vi "StateDrivebase.vi"(1 "Master State":string) -> ()   [LabVIEW 2019]
doc: "This VI performs all of the calculations and decisions related to the swerve drive. Driver profiles are tuned from this front panel."
uses:
  <vilib>/Rock Robotics/WPI/DriverStation/WPI_DriverStationRobotMode2.ctl
  dsinstructions.vi
  constants.vi
  dsdata.vi
  sensors.vi
  outputs.vi
panel:
  in  "PID Tuning Heading Lock":T1={"Kp"=0.00045, "Ki"=0.0, "Kd"=0.0, "N-Diff"=3, "N-Int"=10, "Int Error Window"=90.0, "Max Ouput"=1.0, "Min Output"=-1.0, "Square Derivative"=FALSE, "N-Prop"=5} {"N-Prop" min=1; "Int Error Window" min=0.0; "N-Int" min=2; "N-Diff" min=2; "Kd" min=0.0; "Ki" min=0.0; "Kp" min=0.0}
  in  "Driver Profiles":T2(array[cluster])=[{"Strafe Deadband"=0.08, "Strafe Scaling"=2.0, "Strafe Maximum"=1.0, "Rotation Deadband"=0.15, "Rotation Scaling"=2.5, "Rotation Maximum"=1.0}, {"Strafe Deadband"=0.08, "Strafe Scaling"=2.0, "Strafe Maximum"=1.0, "Rotation Deadband"=0.15, "Rotation Scaling"=2.5, "Rotation Maximum"=1.0}, {"Strafe Deadband"=0.08, "Strafe Scaling"=2.0, "Strafe Maximum"=1.0, "Rotation Deadband"=0.15, "Rotation Scaling"=2.5, "Rotation Maximum"=1.0}, {"Strafe Deadband"=0.08, "Strafe Scaling"=2.0, "Strafe Maximum"=1.0, "Rotation Deadband"=0.03, "Rotation Scaling"=2.5, "Rotation Maximum"=1.0}, {"Strafe Deadband"=0.08, "Strafe Scaling"=2.0, "Strafe Maximum"=1.0, "Rotation Deadband"=0.15, "Rotation Scaling"=2.5, "Rotation Maximum"=1.0}, {"Strafe Deadband"=0.08, "Strafe Scaling"=2.0, "Strafe Maximum"=1.0, "Rotation Deadband"=0.15, "Rotation Scaling"=2.5, "Rotation Maximum"=1.0}, {"Strafe Deadband"=0.08, "Strafe Scaling"=2.0, "Strafe Maximum"=0.5, "Rotation Deadband"=0.15, "Rotation Scaling"=2.5, "Rotation Maximum"=0.3}] {"Rotation Maximum" min=0.3 max=1.0 scale=0.3..1.0; "Rotation Scaling" min=1.0 max=4.0 scale=1.0..4.0; "Rotation Deadband" min=0.0 max=0.25 scale=0.0..0.25; "Strafe Maximum" min=0.3 max=1.0 scale=0.3..1.0; "Strafe Scaling" min=1.0 max=4.0 scale=1.0..4.0; "Strafe Deadband" min=0.0 max=0.25 scale=0.0..0.25}
  in  "Deceleration Hysteresis (ms)":u32=1
  out "Heading Control":bool
  in  "Heading Lock Strafe Deadband (ft/s)":dbl=3.0
  in  "Manually Disable Heading Lock":bool
  in  "PID Tuning Feeder Station":T3={"Kp"=0.0045, "Ki"=0.01, "Kd"=0.0002, "N-Diff"=10, "N-Int"=10, "Int Error Window"=30.0, "Max Ouput"=1.0, "Min Output"=-1.0} {"Int Error Window" min=0.0; "N-Int" min=2; "N-Diff" min=2; "Kd" min=0.0; "Ki" min=0.0; "Kp" min=0.0}
  out "Heading Controller Summary":T4(graph)
  in  "PID Tuning Auto Targeting":T3={"Kp"=0.0045, "Ki"=0.01, "Kd"=0.0002, "N-Diff"=10, "N-Int"=10, "Int Error Window"=30.0, "Max Ouput"=1.0, "Min Output"=-1.0} {"Int Error Window" min=0.0; "N-Int" min=2; "N-Diff" min=2; "Kd" min=0.0; "Ki" min=0.0; "Kp" min=0.0}
  in  "Manual Fudge Factor (deg)":dbl=5.0
  in  "Plot Heading PID":bool
  in  "Sync Driver Profile":bool
  out "Selected Driver":string
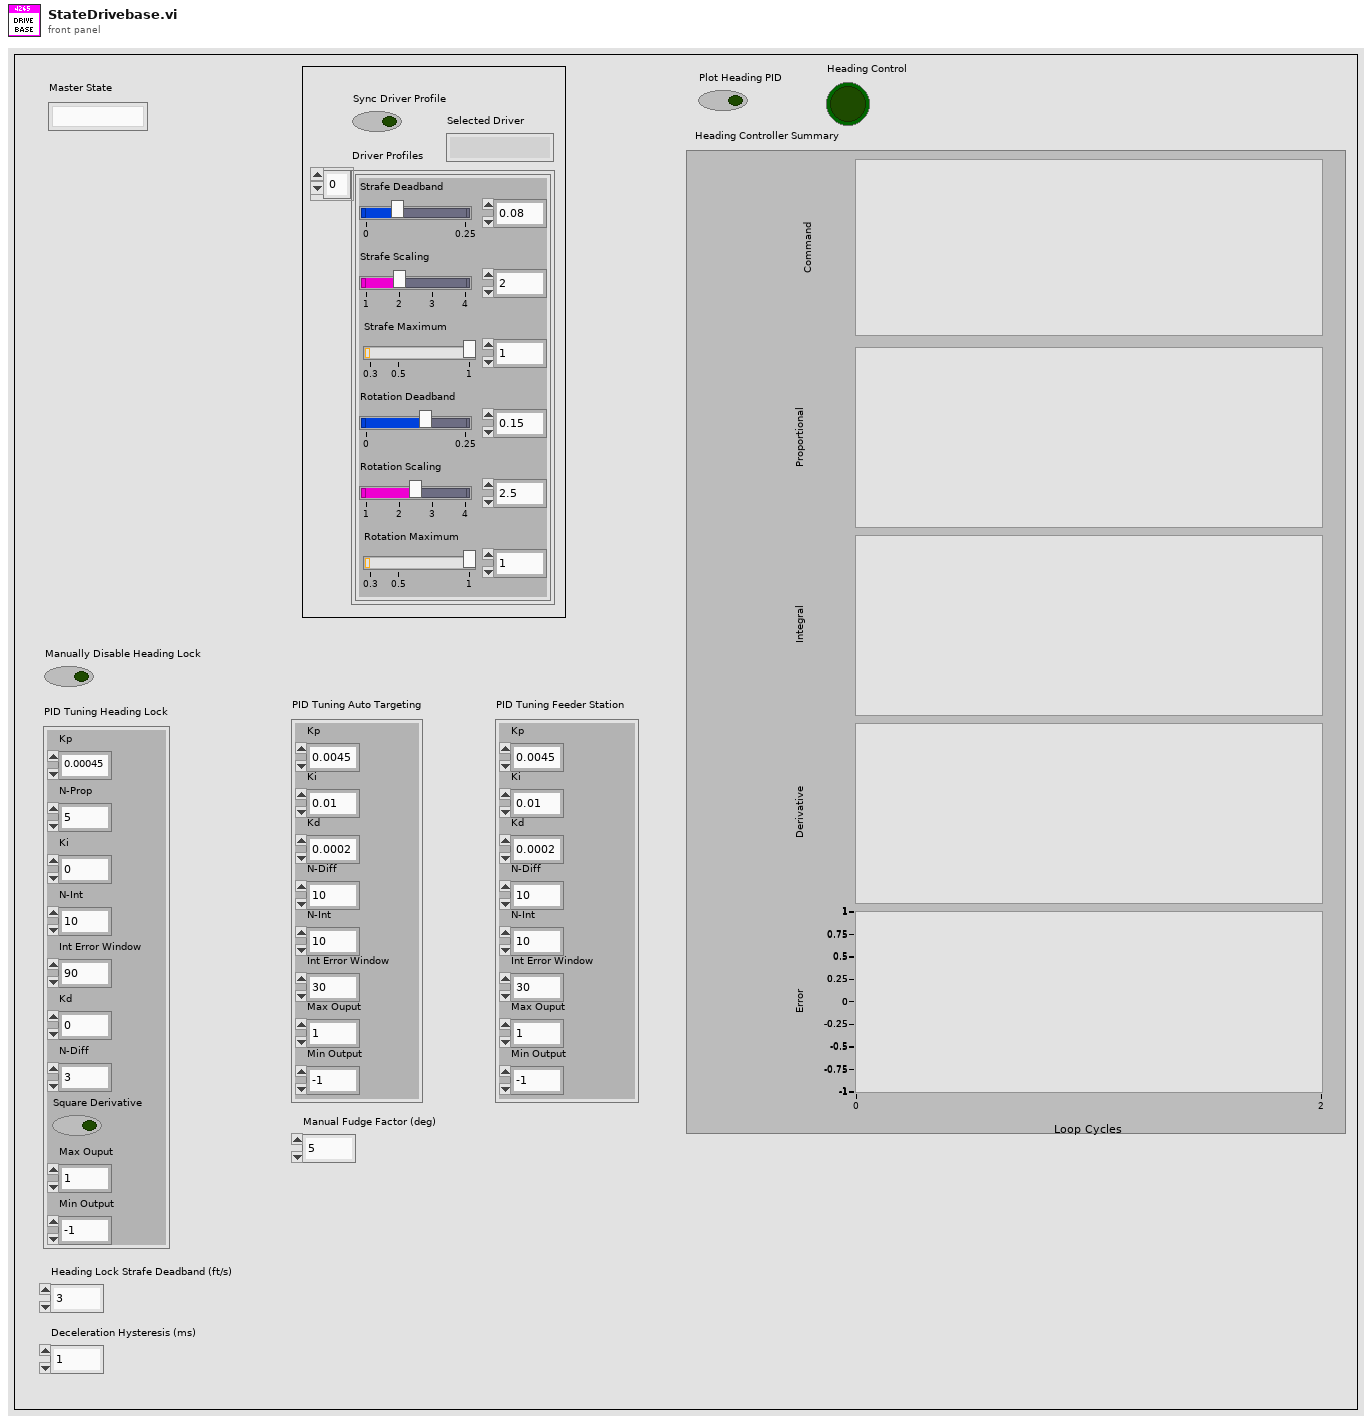
[diagram p1: front panel]
types:
  T1 = cluster{"Kp":dbl, "Ki":dbl, "Kd":dbl, "N-Diff":i32, "N-Int":i32, "Int Error Window":dbl, "Max Ouput":dbl, "Min Output":dbl, "Square Derivative":bool, "N-Prop":i32}
  T2 = cluster{"Strafe Deadband":dbl, "Strafe Scaling":dbl, "Strafe Maximum":dbl, "Rotation Deadband":dbl, "Rotation Scaling":dbl, "Rotation Maximum":dbl}[]
  T3 = cluster{"Kp":dbl, "Ki":dbl, "Kd":dbl, "N-Diff":i32, "N-Int":i32, "Int Error Window":dbl, "Max Ouput":dbl, "Min Output":dbl}
  T4 = cluster{"Command":dbl, "Proportional":dbl, "Integral":dbl, "Derivative":dbl, "Goal":dbl}
  T5 = enum16{"Driver Control", "Auto Targeting", "Feeder Station"}
  T6 = typedef "WPI_DriverStationRobotMode2.ctl" = enum16{"Autonomous Disabled", "Autonomous Enabled", "Teleop Disabled", "Teleop Enabled", "Disconnected", "Finish", "Test Disabled", "Test Enabled", "Emergency Stopped"}
  T7 = cluster{"Strafe Deadband":dbl, "Strafe Scaling":dbl, "Strafe Maximum":dbl, "Rotation Deadband":dbl, "Rotation Scaling":dbl, "Rotation Maximum":dbl}
  T8 = enum16{"Center", "Module 0", "Module 1", "Module 2", "Module 3"}
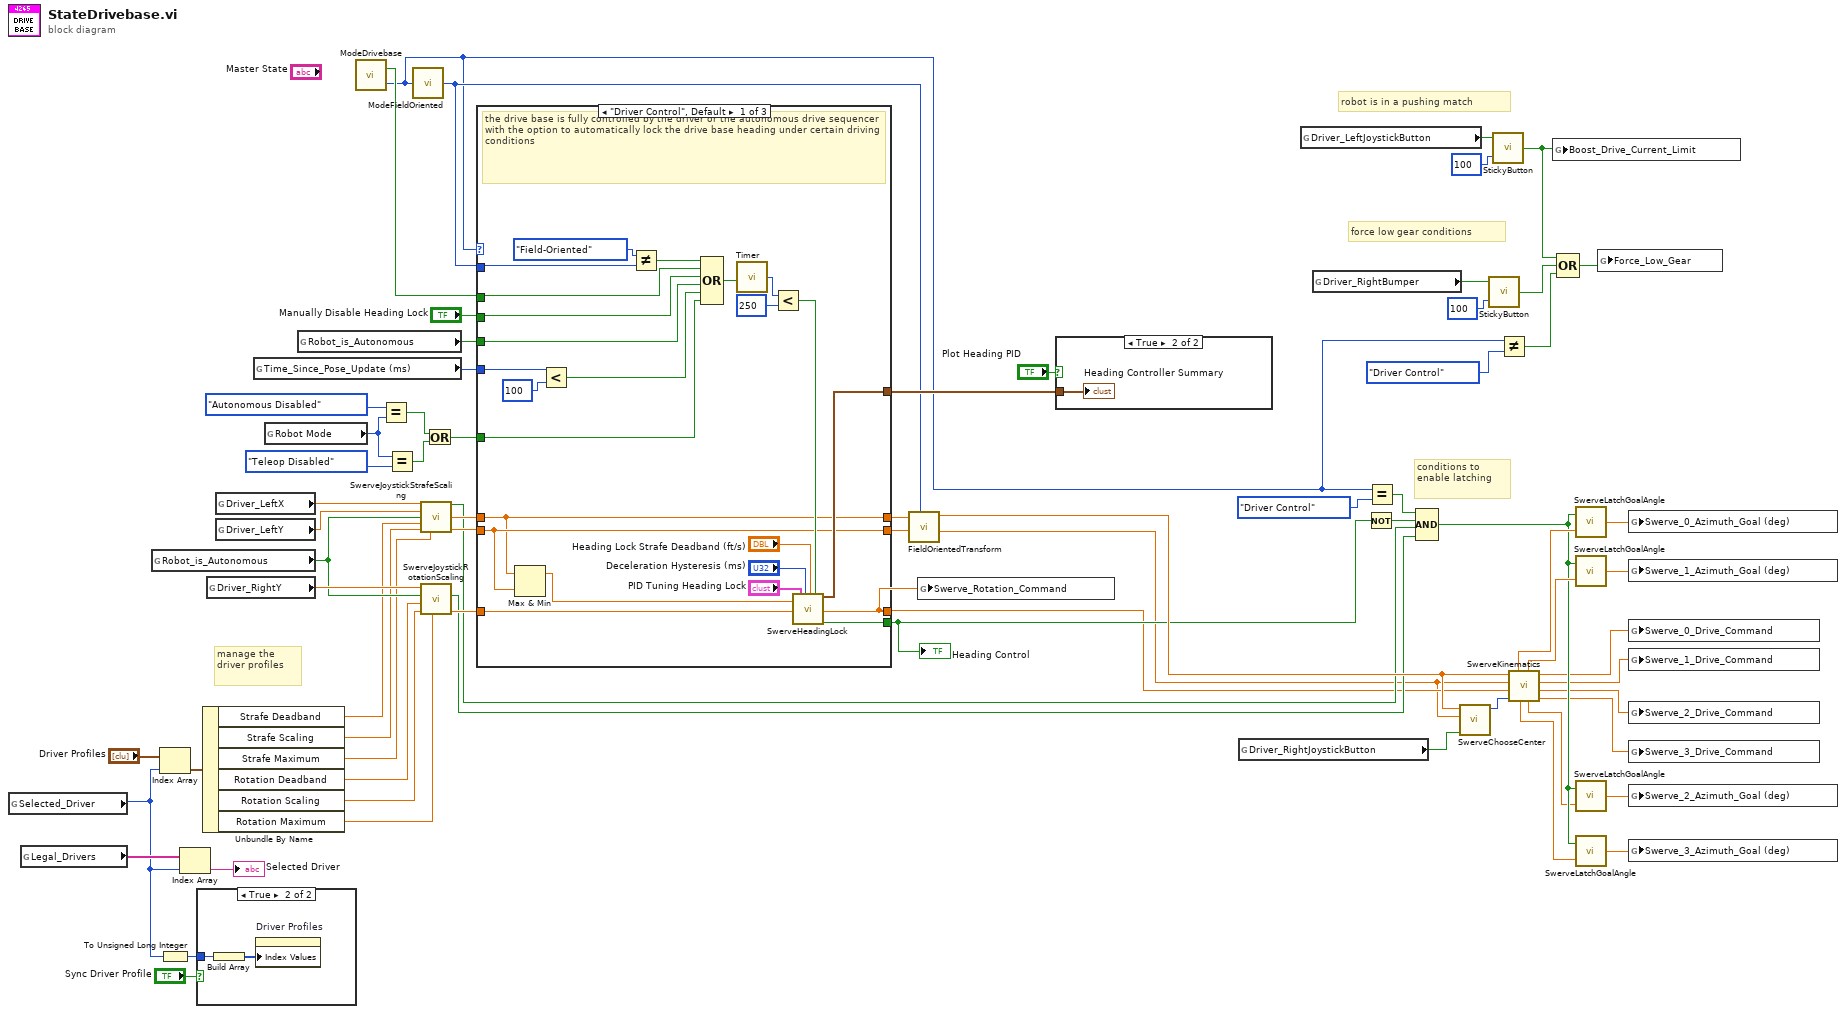
[diagram p0: block diagram]
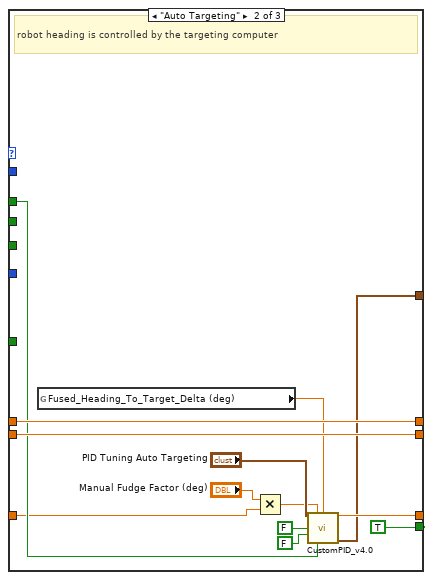
[diagram p3: hidden frame]
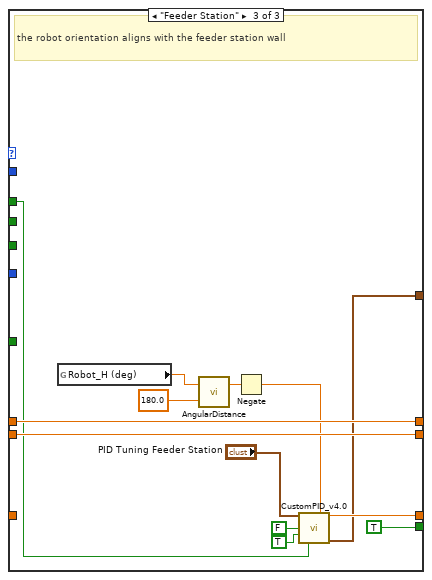
[diagram p4: hidden frame]
diagram:
  # "force low gear conditions"
  # "robot is in a pushing match"
  # "conditions to\nenable latching"
  # "manage the\ndriver profiles"
  n1 = global read "dsdata.vi" "Selected_Driver"() -> (w31:i32)
  n2 = global read "constants.vi" "Legal_Drivers"() -> (w63:string[])
  n3 = global read "dsdata.vi" "Robot_is_Autonomous"() -> (w43:bool)
  n4 = Index Array(array="Driver Profiles", index=w31) -> (element=w30:T7)
  n5 = To Unsigned Long Integer(number=w31) -> (unsigned 32bit integer=w65:u32)
  n6 = Index Array(array=w63, index=w31) -> (element=→"Selected Driver":string)
  n7 = case shown="True" "Sync Driver Profile" {
    tunnel: w65 -> [_ w71]
    frame False {
    }
    frame True {
      n8 = Build Array(w71) -> (w70:u32[])
      n9 = property on="Driver Profiles" class="Arr (strict)"("Index Values"=w70) -> ()  [unwired: 2 in, 2 out]
    }
  }
  n10 = Unbundle By Name(w30) -> ("Strafe Deadband"=w29:dbl, "Strafe Scaling"=w28:dbl, "Strafe Maximum"=w9:dbl, "Rotation Deadband"=w12:dbl, "Rotation Scaling"=w11:dbl, "Rotation Maximum"=w10:dbl)
  n11 = global read "dsinstructions.vi" "Driver_RightY"() -> (w44:dbl)
  n12 = global read "dsinstructions.vi" "Driver_LeftX"() -> (w49:dbl)
  n13 = global read "dsinstructions.vi" "Driver_LeftY"() -> (w48:dbl)
  n14 = global read "sensors.vi" "Time_Since_Pose_Update (ms)"() -> (w58:u32)
  n15 = global read "dsdata.vi" "Robot Mode"() -> (w18:T6)
  n16 = global read "dsdata.vi" "Robot_is_Autonomous"() -> (w57:bool)
  n17 = call "ModeDrivebase.vi"() -> ("Drive Mode Change"=w55:bool, "Drive Mode"=w1:T5)  [unwired: 1 in]
  n18 = Equal?(x=WPI_DriverStationRobotMode2."Autonomous Disabled" ("Robot Mode"), y=w18) -> (x = y?=w16:bool)
  n19 = Equal?(x=w18, y=WPI_DriverStationRobotMode2."Teleop Disabled" ("Robot Mode")) -> (x = y?=w15:bool)
  n20 = call "ModeFieldOriented.vi"("Drive Mode"=w1) -> ("Orientation Mode"=w33:enum16{"Robot-Oriented", "Field-Oriented"})
  n21 = call "SwerveJoystickStrafeScaling.vi"("Raw Joystick X"=w49, "Raw Joystick Y"=w48, "Auto Control"=w43, "Strafe Deadband"=w29, "Strafe Scaling"=w28, "Strafe Maximum"=w9) -> ("In Deadband"=w39:bool, "Scaled Joystick X"=w47:dbl, "Scaled Joystick Y"=w46:dbl)  [unwired: 7 in]
  n22 = call "SwerveJoystickRotationScaling.vi"("Rotation Maximum"=w10, "Rotation Scaling"=w11, "Rotation Deadband"=w12, "Auto Control"=w43, "Raw Joystick Rotation"=w44) -> ("Scaled Joystick Rotation"=w45:dbl, "In Deadband"=w40:bool)  [unwired: 4 in]
  n23 = Or(x=w16, y=w15) -> (x .or. y?=w14:bool)
  n24 = case shown="\"Driver Control\", Default" w1 {
    tunnel: [w74 w107 w119] -> w32
    tunnel: [w73 w108 w117] -> w69
    tunnel: w47 -> [w73 w108 w117]
    tunnel: w46 -> [w74 w107 w119]
    tunnel: w45 -> [w85 w97 _]
    tunnel: [w86 w99 w116] -> w38
    tunnel: [w91 TRUE ("auto rot control") TRUE ("auto rot control")] -> w41
    tunnel: w33 -> [w92 _ _]
    tunnel: w57 -> [w89 _ _]
    tunnel: w55 -> [w83 w102 w112]
    tunnel: w58 -> [w95 _ _]
    tunnel: [w88 w98 w111] -> w56
    tunnel: "Manually Disable Heading Lock" -> [w87 _ _]
    tunnel: w14 -> [w77 _ _]
    frame "Driver Control", Default {
      # "the drive base is fully controlled by the driver or the autonomous drive sequencer with the option to automatically lock the drive base heading under certain driving conditions"
      n25 = Max & Min(x=w73, y=w74) -> (max(x,y)=w72:dbl)  [unwired: 1 out]
      n26 = Less?(x=w95, y=u32 100) -> (x < y?=w90:bool)
      n27 = Not Equal?(x=enum16{"Robot-Oriented", "Field-Oriented"}."Field-Oriented" ("Orientation Mode"), y=w92) -> (x != y?=w82:bool)
      n28 = Compound Arithmetic op=OR(w82, w83, w87, w89, w90, w77) -> (w80:bool)
      n29 = call "Timer.vi"("Reset Timer"=w80) -> ("Time (ms)"=w81:u32)
      n30 = Less?(x=w81, y=u32 250) -> (x < y?=w78:bool)
      n31 = call "SwerveHeadingLock.vi"("Max Driver Translation Joystick"=w72, "Driver Rotation Joystick"=w85, "PID Tuning Parameters"="PID Tuning Heading Lock", "Deceleration Hysteresis (ms)"="Deceleration Hysteresis (ms)", "Heading Lock Strafe Deadband (ft/s)"="Heading Lock Strafe Deadband (ft/s)", "External Disables"=w78) -> ("Controller Summary"=w88:T4, "Joystick Rotation"=w86:dbl, "Heading Lock"=w91:bool)  [unwired: 11 in]
    }
    frame "Auto Targeting" {
      # "robot heading is controlled by the targeting computer"
      n32 = global read "sensors.vi" "Fused_Heading_To_Target_Delta (deg)"() -> (w103:dbl)
      n33 = Multiply(x="Manual Fudge Factor (deg)", y=w97) -> (x*y=w104:dbl)
      n34 = call "CustomPID_v4.0.vi"("PID Tuning Parameters"="PID Tuning Auto Targeting", "Goal"=w104, "Process Variable"=w103, "Reset on Goal Change ?"=FALSE, "Use Custom Error Calculation ?"=FALSE, "Reinit"=w102) -> ("Command"=w99:dbl, "Controller Summary"=w98:T4)  [unwired: 6 in, 2 out]
    }
    frame "Feeder Station" {
      # "the robot orientation aligns with the feeder station wall"
      n35 = global read "sensors.vi" "Robot_H (deg)"() -> (w121:dbl)
      n36 = call "AngularDistance.vi"("Goal Angle (deg) [0,360]"=180.0, "Current Angle (deg) [-Inf,+Inf]"=w121) -> ("Signed Angular Distance (deg) [-180,+180]"=w110:dbl)  [unwired: 1 out]
      n37 = Negate(x=w110) -> (-x=w109:dbl)
      n38 = call "CustomPID_v4.0.vi"("PID Tuning Parameters"="PID Tuning Feeder Station", "Custom Error Calculation"=w109, "Reset on Goal Change ?"=FALSE, "Use Custom Error Calculation ?"=TRUE, "Reinit"=w112) -> ("Command"=w116:dbl, "Controller Summary"=w111:T4)  [unwired: 7 in, 2 out]
    }
  }
  "Heading Control" <- w41
  n39 = call "FieldOrientedTransform.vi"("Orientation Mode"=w33, "Joystick Y"=w32, "Joystick X"=w69) -> ("Joystick Y'"=w34:dbl, "Joystick X'"=w42:dbl)  [unwired: 7 in]
  n40 = global write "outputs.vi" "Swerve_Rotation_Command"(w38) -> ()
  n41 = case shown="True" "Plot Heading PID" {
    tunnel: w56 -> [_ w122]
    frame False {
    }
    frame True {
      "Heading Controller Summary" <- w122
    }
  }
  n42 = global read "dsinstructions.vi" "Driver_RightJoystickButton"() -> (w54:bool)
  n43 = global read "dsinstructions.vi" "Driver_LeftJoystickButton"() -> (w51:bool)
  n44 = global read "dsinstructions.vi" "Driver_RightBumper"() -> (w8:bool)
  n45 = Not(x=w41) -> (.not. x?=w37:bool)
  n46 = Equal?(x=w1, y=T5."Driver Control" ("x")) -> (x = y?=w36:bool)
  n47 = Compound Arithmetic op=AND(w36, w37, w39, w40) -> (w61:bool)
  n48 = call "SwerveChooseCenter.vi"("Defensive Driving Trigger"=w54, "Joystick Y"=w34, "Joystick X"=w42) -> ("Center Choice"=w53:T8)  [unwired: 6 in]
  n49 = call "StickyButton.vi"("Time threshold (ms)"=u32 100 ("y"), "Button Input"=w8) -> ("Sticky Button"=w5:bool)
  n50 = call "StickyButton.vi"("Time threshold (ms)"=u32 100 ("y"), "Button Input"=w51) -> ("Sticky Button"=w6:bool)
  n51 = Not Equal?(x=w1, y=T5."Driver Control") -> (x != y?=w2:bool)
  n52 = call "SwerveKinematics.vi"("Rotation Center Choice"=w53, "Joystick Rotation"=w38, "Joystick Y"=w34, "Joystick X"=w42) -> ("Module 3 Velocity Command (ul)"=w24:dbl, "Module 2 Velocity Command (ul)"=w25:dbl, "Module 1 Velocity Command (ul)"=w26:dbl, "Module 0 Velocity Command (ul)"=w27:dbl, "Module 2 Angle (deg)"=w60:dbl, "Module 1 Angle (deg)"=w67:dbl, "Module 3 Angle (deg)"=w59:dbl, "Module 0 Angle (deg)"=w68:dbl)
  n53 = global write "outputs.vi" "Boost_Drive_Current_Limit"(w6) -> ()
  n54 = Compound Arithmetic op=OR(w6, w5, w2) -> (w4:bool)
  n55 = call "SwerveLatchGoalAngle.vi"("Raw Goal Angle"=w68, "In Deadband"=w61) -> ("Latched Goal Angle"=w23:dbl)
  n56 = call "SwerveLatchGoalAngle.vi"("Raw Goal Angle"=w67, "In Deadband"=w61) -> ("Latched Goal Angle"=w22:dbl)
  n57 = call "SwerveLatchGoalAngle.vi"("Raw Goal Angle"=w60, "In Deadband"=w61) -> ("Latched Goal Angle"=w21:dbl)
  n58 = call "SwerveLatchGoalAngle.vi"("Raw Goal Angle"=w59, "In Deadband"=w61) -> ("Latched Goal Angle"=w20:dbl)
  n59 = global write "outputs.vi" "Force_Low_Gear"(w4) -> ()
  n60 = global write "outputs.vi" "Swerve_0_Azimuth_Goal (deg)"(w23) -> ()
  n61 = global write "outputs.vi" "Swerve_1_Azimuth_Goal (deg)"(w22) -> ()
  n62 = global write "outputs.vi" "Swerve_0_Drive_Command"(w27) -> ()
  n63 = global write "outputs.vi" "Swerve_1_Drive_Command"(w26) -> ()
  n64 = global write "outputs.vi" "Swerve_2_Drive_Command"(w25) -> ()
  n65 = global write "outputs.vi" "Swerve_3_Drive_Command"(w24) -> ()
  n66 = global write "outputs.vi" "Swerve_2_Azimuth_Goal (deg)"(w21) -> ()
  n67 = global write "outputs.vi" "Swerve_3_Azimuth_Goal (deg)"(w20) -> ()
